vi "Perform Action.vi"(8 "error in":errorcluster, 10 "Input":variant, 11 "CFG Base in":refnum<class "CFG Base.lvclass">=refnum) -> (0 "error out":errorcluster, 2 "Output":variant, 3 "CFG Base out":refnum<class "CFG Base.lvclass">)   [LabVIEW 2023, in "HAL.lvlib" / "CFG Base.lvclass"]
uses:
  CFG Base.lvclass
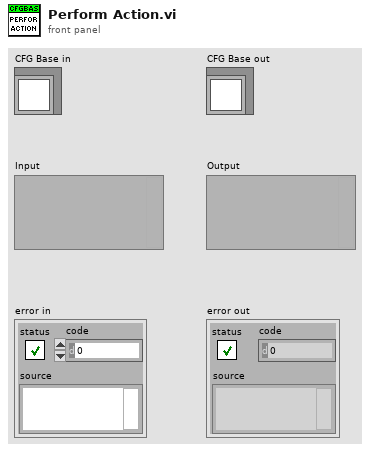
[diagram p1: front panel]
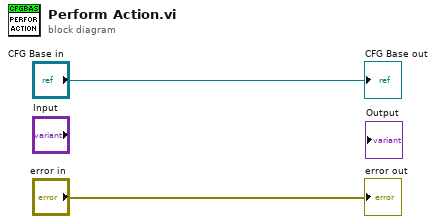
[diagram p0: block diagram]
diagram:
  "error out" <- "error in"
  "CFG Base out" <- "CFG Base in"
